vi "Store Actors.vi"(8 "error in (no error)":errorcluster, 9 "Actor Paths":path[](array[path]), 10 "Actors":string[](array[string]), 11 "Actor Store in":refnum<class "Actor Store.lvclass">) -> (0 "error out":errorcluster, 3 "Actor Store out":refnum<class "Actor Store.lvclass">)   [LabVIEW 2023, in "Add Async Methods Actor.lvlib" / "Actor Store.lvclass"]
uses:
  Actor Store.lvclass
  <vilib>/Utility/error.llb/Error Cluster From Error Code.vi
  <vilib>/ErrorRing/Error Ring.xnode
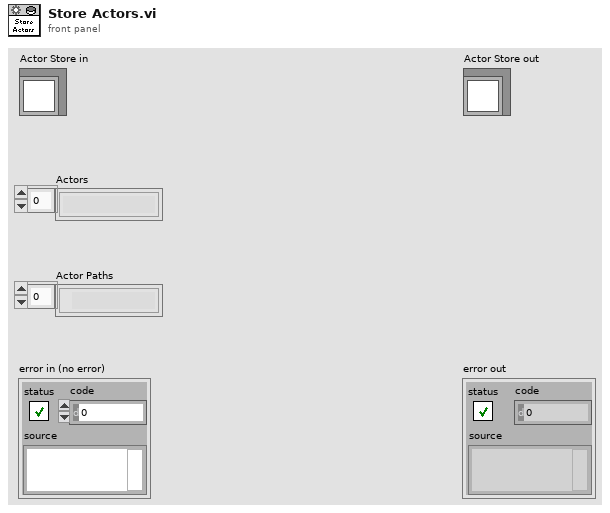
[diagram p1: front panel]
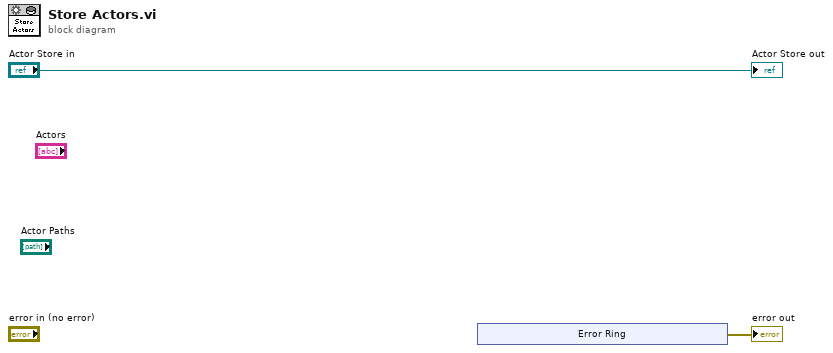
[diagram p0: block diagram]
diagram:
  n1 = xnode "Error Ring"() -> ("error out"=→"error out":errorcluster)
  "Actor Store out" <- "Actor Store in"
